vi "Set Color by BaseColor and Alpha.vi"(8 "error in (no error)":errorcluster caption="错误输入（无错误）", 10 "alpha":i32, 11 "Color":refnum<k24>) -> (0 "error out":errorcluster caption="错误输出", 3 "FromArgb":refnum<k24>)   [LabVIEW 2012, in "Color.lvclass"]
uses:
  Color.lvclass
  System.Drawing
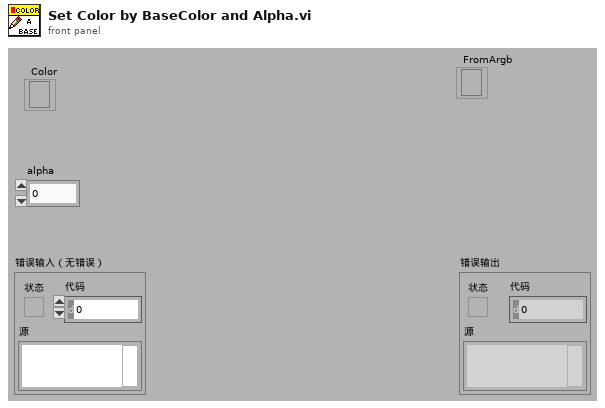
[diagram p1: front panel]
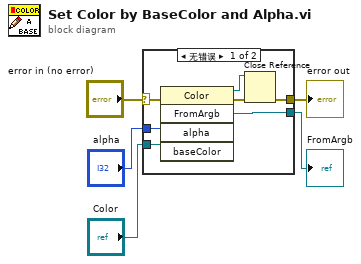
[diagram p0: block diagram]
diagram:
  n1 = case shown="无错误" "error in (no error)" {
    selector: "error in (no error)" -> [w10 w13]
    tunnel: [w9 w13] -> w4
    tunnel: "Color" -> [w12 _]
    tunnel: "alpha" -> [w11 _]
    tunnel: [w6 _] -> w1
    frame No Error {
      n2 = invoke class="Color" method="FromArgb"(error in=w10, "alpha"=w11, "baseColor"=w12) -> (reference out=w8:refnum<k24>, error out=w7:errorcluster, "FromArgb"=w6:refnum<k24>)  [unwired: 2 in, 2 out]
      n3 = Close Reference(reference=w8, error in (no error)=w7) -> (error out=w9:errorcluster)
    }
    frame Error {
    }
  }
  "error out" <- w4
  "FromArgb" <- w1
